vi "DataLib.unpack event data.vi"(1 "serviceData":T1, 2 "descriptor":string, 5 "error in (no error)":errorcluster) -> (15 "headerID":dbl, 16 "timestamp":dbl, 17 "eventID":i32, 18 "subEventData":T1, 19 "error out":errorcluster)   [LabVIEW 2014, in "DataLib.lvlib"]
doc: "This routine can be used to unpack data received by the DIM service \"EVENTBUILDERNAME_eventData\"."
uses:
  DataLib.lvlib
  CS_Core/CSSystem/CoreDefs/CoreDefs.rawDataType.ctl
  CS_Core/CSSystem/CoreLib/CoreLib.lvlib
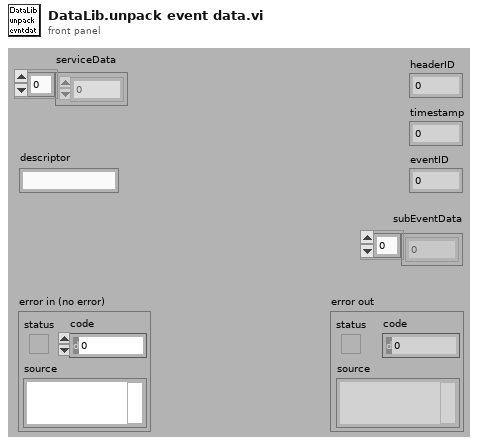
[diagram p1: front panel]
types:
  T1 = typedef "CoreDefs.rawDataType.ctl" = i8[]
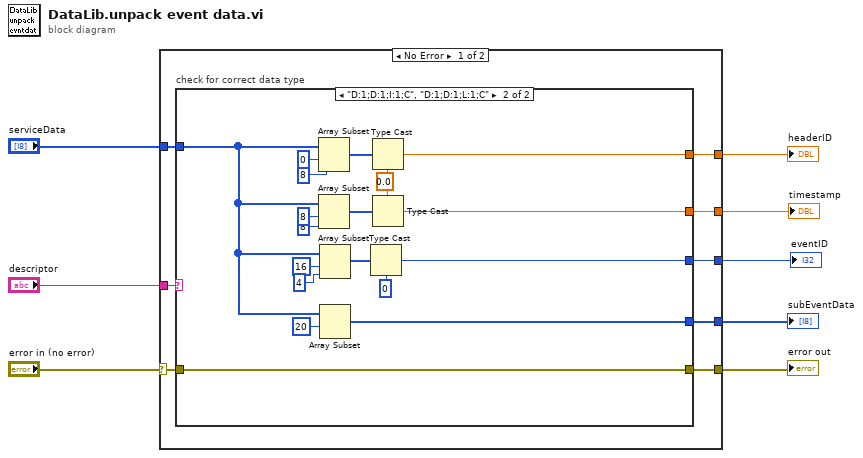
[diagram p0: block diagram]
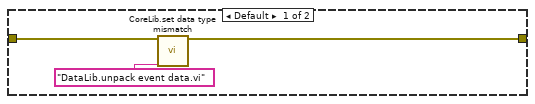
[diagram p2: hidden frame]
diagram:
  n1 = case shown="No Error" "error in (no error)" {
    selector: "error in (no error)" -> [w12 w38]
    tunnel: [w16 _] -> w8
    tunnel: "descriptor" -> [w15 _]
    tunnel: "serviceData" -> [w14 _]
    tunnel: [w13 w38] -> w5
    tunnel: [w11 _] -> w3
    tunnel: [w10 _] -> w2
    tunnel: [w9 _] -> w1
    frame No Error {
      n2 = case "check for correct data type" shown="\"D:1;D:1;I:1;C\", \"D:1;D:1;L:1;C\"" w15 {
        tunnel: [_ w29] -> w16
        tunnel: w14 -> [_ w22]
        tunnel: [w19 w28] -> w13
        tunnel: w12 -> [w18 w28]
        tunnel: [_ w26] -> w11
        tunnel: [_ w24] -> w10
        tunnel: [_ w20] -> w9
        frame Default {
          n3 = call "CoreLib.set data type mismatch.vi"("error in (no error)"=w18, "error source"="DataLib.unpack event data.vi") -> ("error out"=w19:errorcluster)  [unwired: 17 in]
        }
        frame "D:1;D:1;I:1;C", "D:1;D:1;L:1;C" {
          w27 = 0.0
          n4 = Array Subset(array=w22, index=0, length=8) -> (w35:T1)
          n5 = Array Subset(array=w22, index=8, length=8) -> (w32:T1)
          n6 = Array Subset(array=w22, index=16, length=4) -> (w30:T1)
          n7 = Array Subset(array=w22, index=20) -> (w20:T1)  [unwired: 1 in]
          n8 = Type Cast(type=0, x=w30) -> (*(type *) &x=w24:i32)
          n9 = Type Cast(type=w27, x=w35) -> (*(type *) &x=w29:dbl)
          n10 = Type Cast(type=w27, x=w32) -> (*(type *) &x=w26:dbl)
        }
      }
    }
    frame Error {
    }
  }
  "headerID" <- w8
  "error out" <- w5
  "timestamp" <- w3
  "eventID" <- w2
  "subEventData" <- w1
